vi "MAIN - Car Wash.vi"() -> ()   [LabVIEW 2015, in "Car Wash.lvlib"]
uses:
  Car Wash.lvlib
  Components/State Declaration.ctl
  Components/System Trigger.ctl
  Components/System Trigger Element.ctl
  <vilib>/Utility/error.llb/DialogTypeEnum.ctl
  Components/AMC/Read Termination Message.vi
  Components/AMC/Update Message Routing Info.vi
  Components/AMC/Create Multiple Messages.vi
  Components/AMC/Create Single Message.vi
  Components/TypeDef - SHIFTER.ctl
  Components/AMC/Globals.vi
  Components/AMC/Send Message.vi
  Components/Dependencies.llb/TLB`_Dependencies.lvlib
  Components/AMC/AMC.lvlib
panel:
  out "Status":string
  in  "Start Wash":bool
  in  "Reset Car":bool
  out "Wash Progress":i32(slide) scale=0.0..6.0
  in  "Giant Blowdryers":bool
  in  "Rinse":bool
  in  "Wax":bool
  in  "Roller Brushes":bool
  in  "Soap":bool
  in  "Pre-Soak":bool
  out "error out":errorcluster
  # "Car Wash"
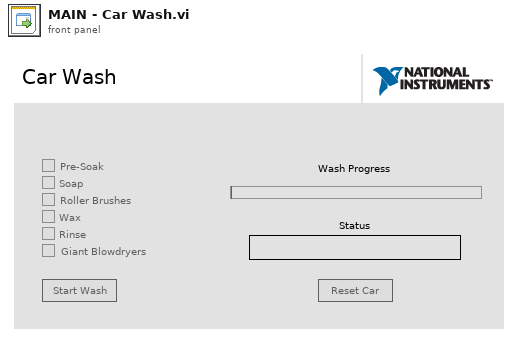
[diagram p1: front panel]
types:
  T1 = typedef "Car Wash.lvlib/System Trigger.ctl" = enum16{"<None>", "Cache User Parameters", "Close Application", "Start Wash", "Reset Car"}
  T2 = typedef "Car Wash.lvlib/State Declaration.ctl" = enum16{"<Startup>", "Idle", "Washing", "<Shutdown>"}
  T3 = enum16{"Clear SR", "Set Display", "Set Shifter", "Initialize Events", "Init Q"}
  T4 = typedef "Car Wash.lvlib/TypeDef - SHIFTER.ctl" = cluster{"State":T2, "User Data":cluster{"Active Item Tag":string, "Pre-Soak":bool, "Soap":bool, "Roller Brushes":bool, "Wax":bool, "Rinse":bool, "Giant Blowdryers":bool}, "Display Data":cluster{"Active Item Tag":string, "Wash Progress":i32, "Status":string}, "User Parameter Controls":refnum<vi>[], "Framework Data":cluster{"Exit Event":T5, "Terminate Error":errorcluster}, "Private Data":cluster{"Active Item Tag":string, "Step Booleans Array":bool[], "Step Names Array":string[], "Wash Done?":bool, "Step Duration":i32}}
  T5 = typedef "Car Wash.lvlib/TLB`_Dependencies.lvlib/Exit Event Ref.ctl" = refnum<user-event>
  T6 = typedef "Car Wash.lvlib/System Trigger Element.ctl" = cluster{"System Triggers":T1, "Trigger Data":variant}
  T7 = typedef "Car Wash.lvlib/AMC.lvlib/Message Queue.ctl" = refnum<queue>
  T8 = enum8{"Enabled", "Disabled", "Disabled and Grayed Out"}
  T9 = typedef "DialogTypeEnum.ctl" = enum16{"no dialog", "OK message", "continue or stop message", "auto error handling dialog", "OK message + warnings", "continue/stop + warnings"}
  T10 = enum32{"Invalid", "Standard", "Closed", "Hidden", "Minimized", "Maximized"}
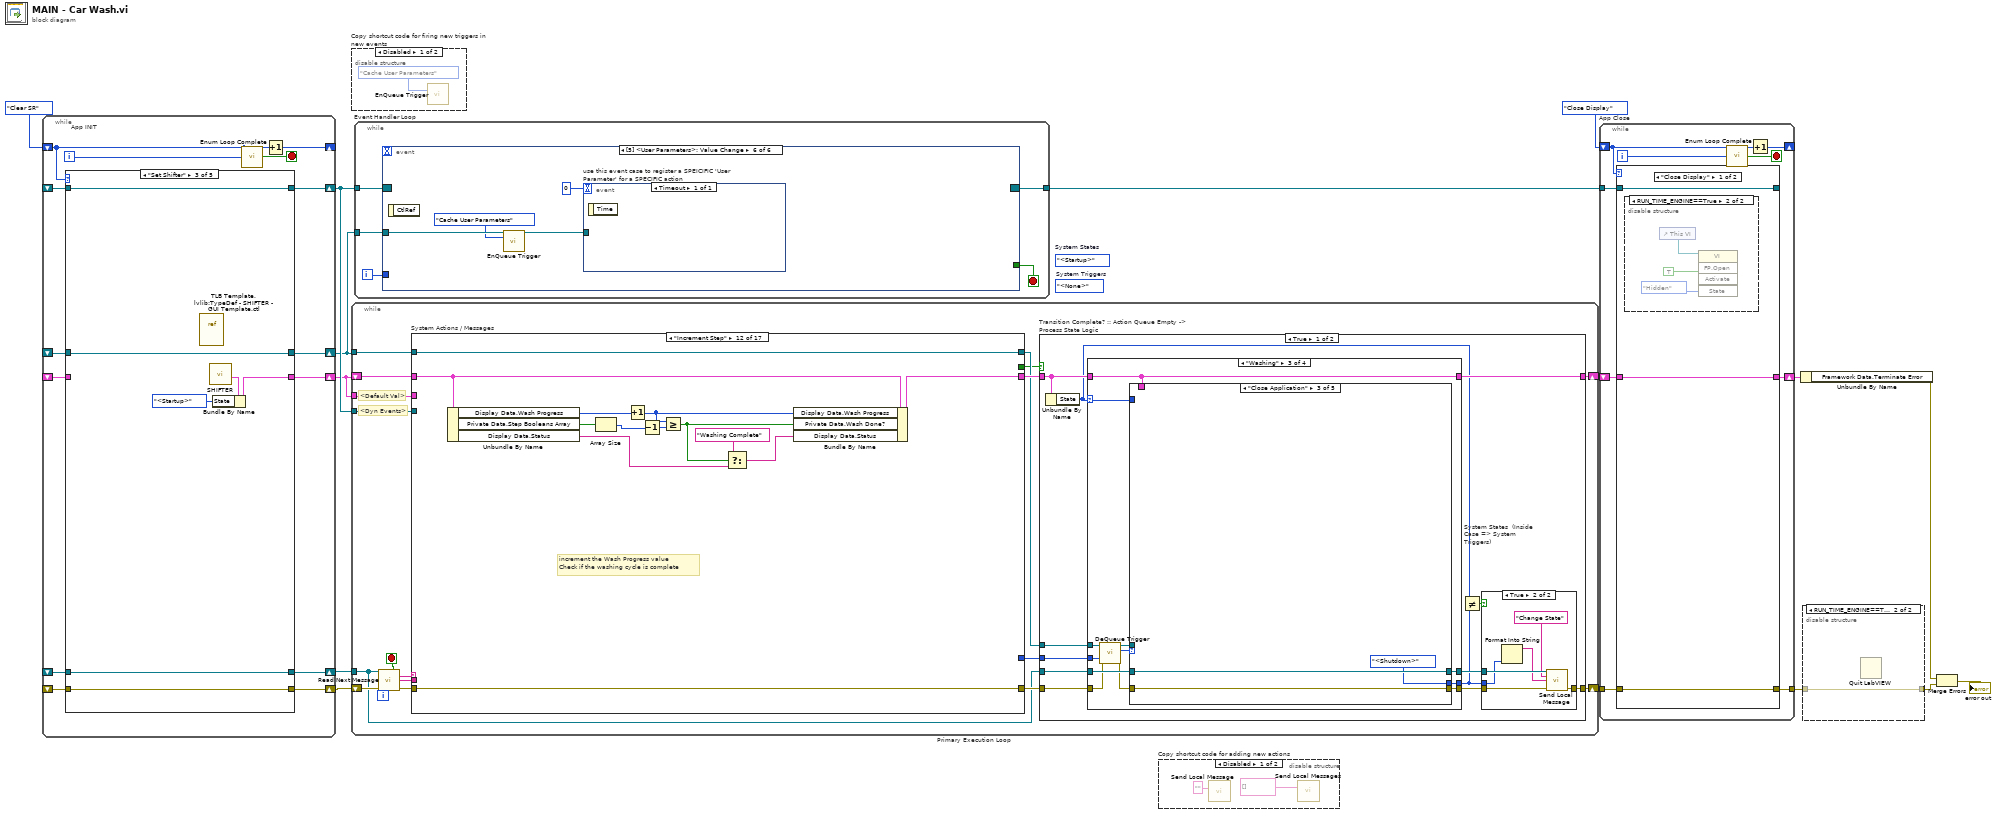
[diagram p0: block diagram]
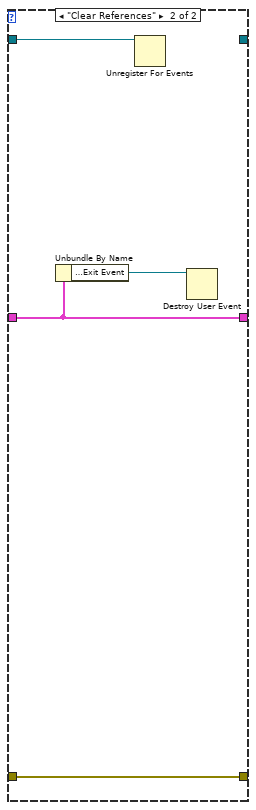
[diagram p6: hidden frame]
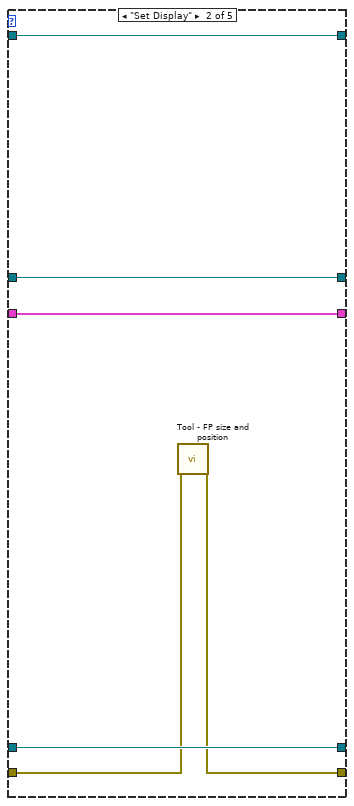
[diagram p8: hidden frame]
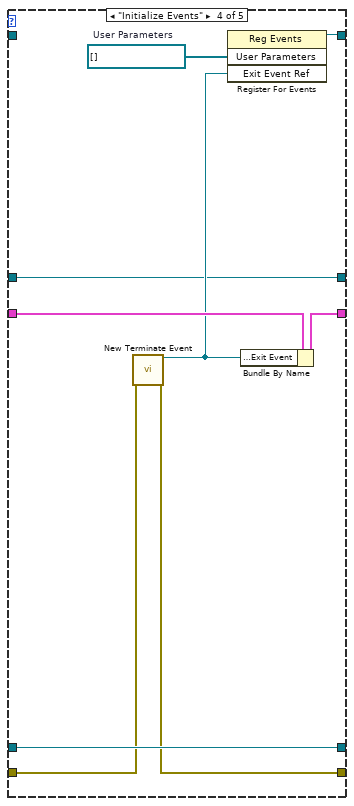
[diagram p9: hidden frame]
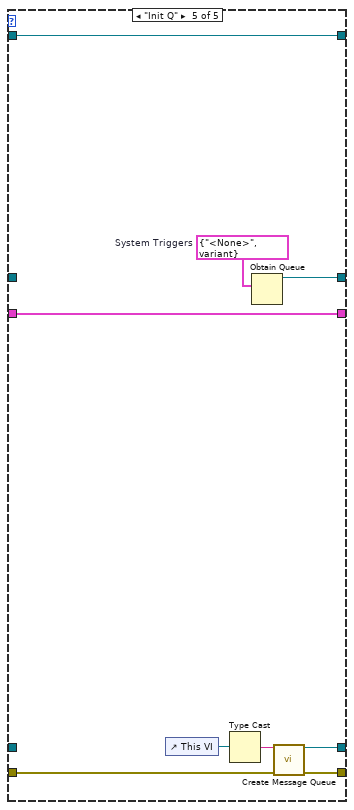
[diagram p10: hidden frame]
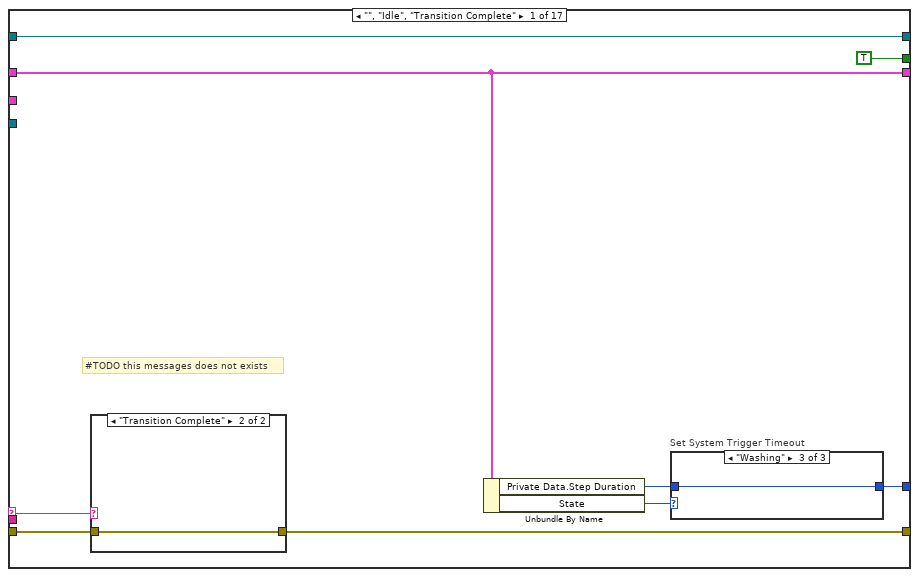
[diagram p11: hidden frame]
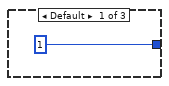
[diagram p13: hidden frame]
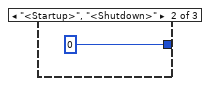
[diagram p14: hidden frame]
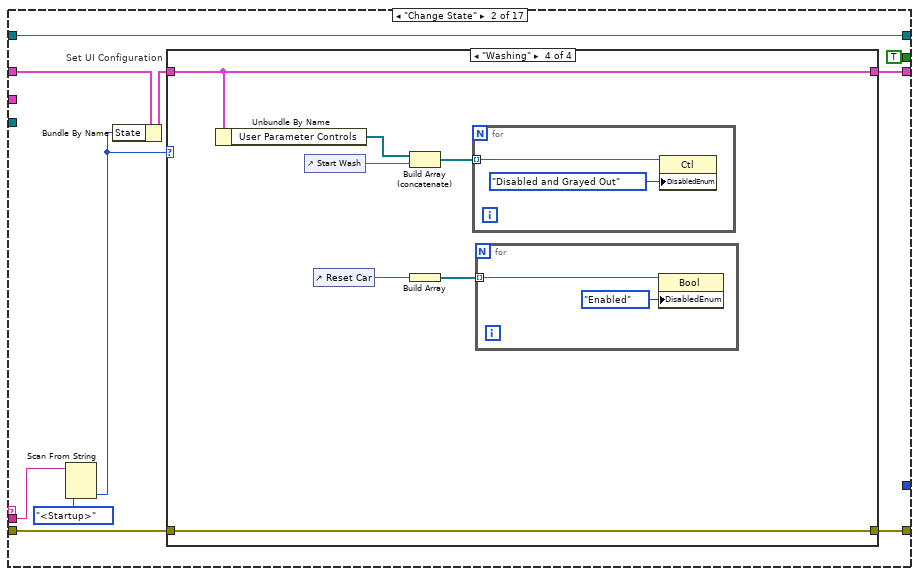
[diagram p15: hidden frame]
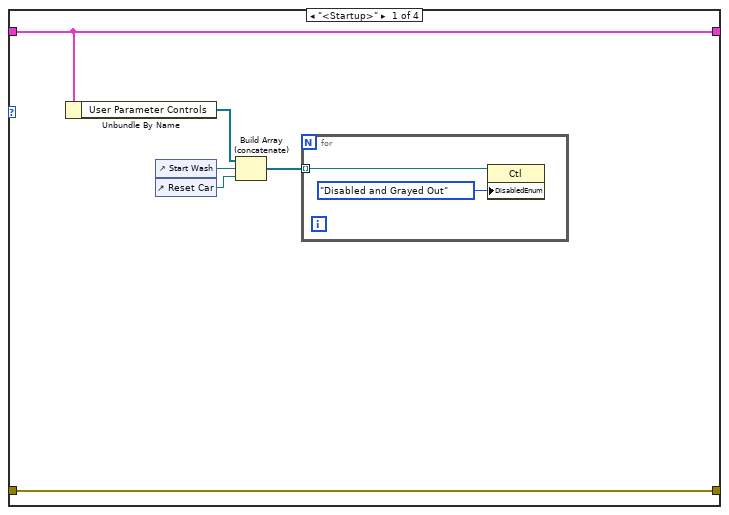
[diagram p16: hidden frame]
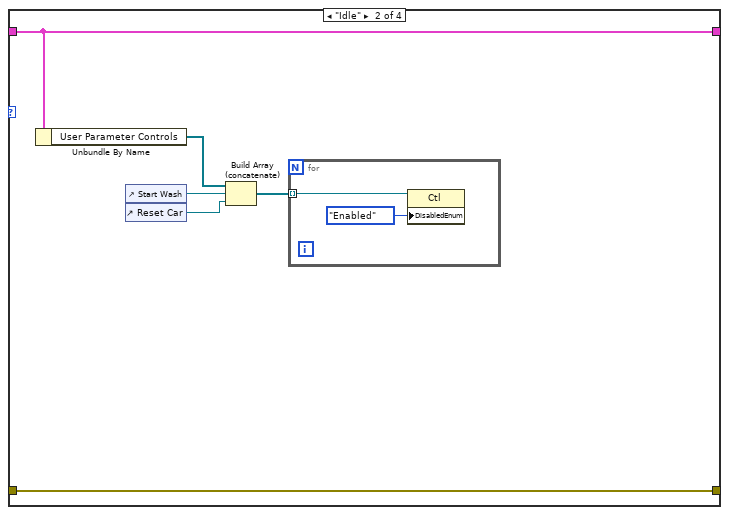
[diagram p17: hidden frame]
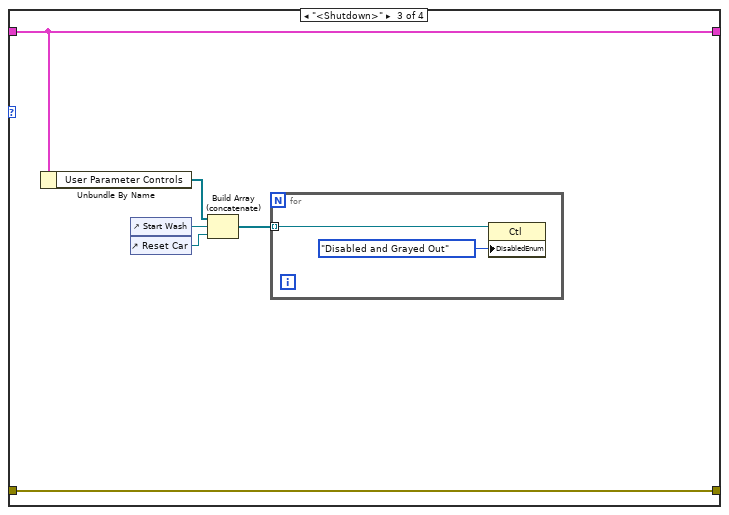
[diagram p18: hidden frame]
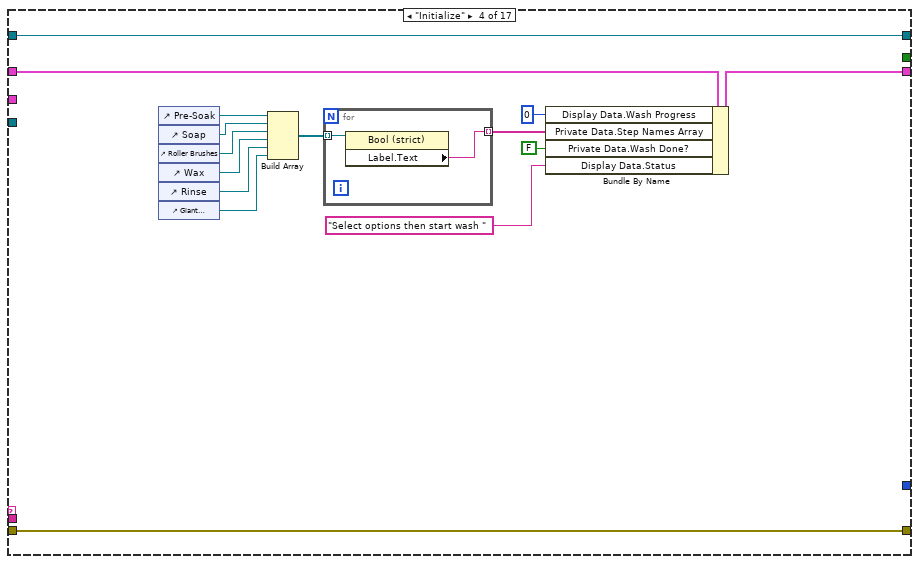
[diagram p20: hidden frame]
diagram:
  (unwired) System_Trigger."<None>"  # System Triggers
  (unwired) State_Declaration."<Startup>"  # System States
  n1 = while "App INIT" {
    shift-right: [w23] -> _
    shift-left: T3."Clear SR" -> [w18]
    shift-right: [w29] -> w9
    shift-left: _ -> [w22]
    shift-right: [w26] -> w8
    shift-left: _ -> [w21]
    shift-right: [w28] -> w11
    shift-left: _ -> [w20]
    shift-right: [w27] -> w1
    shift-left: _ -> [w19]
    shift-right: [w17] -> w2
    shift-left: _ -> [w16]
    i -> [w24]
    stop <- w25 stop-if-true
    n2 = case shown="\"Set Shifter\"" w18 {
      tunnel: [_ w33 w42 w51 w56] -> w29
      tunnel: [_ w31 w41 w44 w55] -> w26
      tunnel: [_ w35 w36 w48 w54] -> w27
      tunnel: [_ w34 w40 w47 w60] -> w28
      tunnel: w22 -> [_ w33 w42 w51 _]
      tunnel: w21 -> [_ w32 w41 w45 w59]
      tunnel: w20 -> [_ w34 w40 _ w60]
      tunnel: w19 -> [_ w35 _ w49 w54]
      tunnel: [_ w30 w39 w43 w58] -> w17
      tunnel: w16 -> [_ w30 w39 w43 _]
      frame "Clear SR" {
      }
      frame "Set Display" {
        n3 = call "Tool - FP size and position.vi"("error in (no error)"=w32) -> ("error out"=w31:errorcluster)  [unwired: 7 in, 11 out]
      }
      frame "Set Shifter" {
        n4 = vi-ref "TLB Template.lvlib:TypeDef - SHIFTER - GUI Template.ctl"() -> ()  [unwired: 1 out]
        n5 = call "SHIFTER.vi"() -> ("SHIFTER DATA"=w37:T4)  [unwired: 15 in]
        n6 = Bundle By Name(cluster=w37, "State"=State_Declaration."<Startup>") -> (w36:T4)
      }
      frame "Initialize Events" {
        w50 = refnum<vi>[] []  # User Parameters
        n7 = call "New Terminate Event.vi"("error in (no error)"=w45) -> ("Exit Event Ref"=w46:T5, "error out"=w44:errorcluster)  [unwired: 13 in]
        n8 = register-events(w50, w46) -> (reference out=w47:refnum<event-registration>)  [unwired: 2 in, 1 out]
        n9 = Bundle By Name(cluster=w49, "Framework Data.Exit Event"=w46) -> (w48:T4)
      }
      frame "Init Q" {
        w57 = T6 {"System Triggers"=enum."<None>", "Trigger Data"=variant}  # System Triggers
        n10 = control-ref of="This VI"() -> (w53:refnum<vi>)
        n11 = Type Cast(x=w53) -> (*(type *) &x=w52:string)  [unwired: 1 in]
        n12 = Obtain Queue(element data type=w57) -> (queue out=w58:refnum<queue>)  [unwired: 4 in, 2 out]
        n13 = call "Create Message Queue.vi"("message queue name"=w52, "error in"=w59) -> ("message queue out"=w56:T7, "error out"=w55:errorcluster)  [unwired: 12 in]
      }
    }
    n14 = call "Enum Loop Complete.vi"("Current State Enum"=w18, "Itteration"=w24) -> ("Loop Complete?"=w25:bool)  [unwired: 13 out]
    n15 = Increment(x=w18) -> (x+1=w23:T3)
  }
  n16 = disable-structure "Copy shortcut code for firing new triggers in new events" shown="Disabled" {
    frame Disabled {
      n17 = call "EnQueue Trigger.vi"("System Triggers"=System_Trigger."Cache User Parameters") -> ()  [unwired: 13 in, 2 out]
    }
    frame Enabled {
    }
  }
  n18 = while "Primary Execution Loop" {
    shift-right: [w68] -> w15
    shift-left: w8 -> [w75]
    shift-right: [w71] -> w14
    shift-left: w1 -> [w78]
    tunnel: w1 -> [w77]
    tunnel: w9 -> [w66]
    tunnel: w11 -> [w76]
    tunnel: w2 -> [w67]
    stop <- w73 stop-if-true
    # "<Dyn Events>"
    # "<Default Val>"
    n19 = call "Read Next Message.vi"("message queue in"=w66, "error in"=w75) -> ("exit process?"=w73:bool, "message name"=w72:string, "message value"=w63:string, "error out"=w74:errorcluster)  [unwired: 6 in, 4 out]
    n20 = case "System Actions / Messages" shown="\"Increment Step\"" w72 {
      selector: w72 -> [w82 _ _ _ _ _ _ _ _ _ _ _ _ _ _ _ w270]
      tunnel: [w81 w97 w140 w154 w169 w180 w183 w191 w198 w201 w212 w229 w233 w236 w241 w264 w274] -> w69
      tunnel: w74 -> [w80 w96 w140 w154 w169 w180 w183 w191 w198 w201 w212 w229 w233 w236 w242 w263 w275]
      tunnel: w78 -> [w83 w93 w139 w150 w168 w173 w182 w193 w196 w199 w205 w225 w231 w235 w239 w267 w276]
      tunnel: w77 -> [_ _ _ _ _ _ _ _ _ _ _ _ _ _ _ _ _]
      tunnel: [w83 w95 w139 w153 w167 w172 w182 w192 w196 w199 w204 w227 w231 w235 w240 w267 w276] -> w70
      tunnel: [w84 _ _ _ _ _ _ _ _ _ _ _ w230 _ _ _ _] -> w62
      tunnel: w76 -> [_ _ _ _ w166 _ _ _ _ _ _ _ _ _ _ _ _]
      tunnel: [w86 w101 w138 w155 w165 w179 w181 w190 w197 w200 w211 w228 w232 w234 w237 w261 w268] -> w65
      tunnel: w67 -> [w86 w101 w138 w155 w165 w179 w181 w190 w197 w200 w211 w228 w232 w234 w237 w261 w268]
      tunnel: [TRUE TRUE _ _ _ _ _ _ _ _ _ _ _ _ _ _ _] -> w64
      tunnel: w63 -> [_ w100 _ _ _ _ _ _ _ _ _ _ _ _ _ _ _]
      frame "", "Idle", "Transition Complete" {
        # "#TODO this messages does not exists"
        n21 = case shown="\"Transition Complete\"" w82 {
          tunnel: [w88 w89] -> w81
          tunnel: w80 -> [w88 w89]
          frame Default {
          }
          frame "Transition Complete" {
          }
        }
        n22 = Unbundle By Name(w83) -> ("Private Data.Step Duration"=w79:i32, "State"=w85:T2)
        n23 = case "Set System Trigger Timeout" shown="\"Washing\"" w85 {
          tunnel: [1 0 w92] -> w84
          tunnel: w79 -> [_ _ w92]
          frame Default {
          }
          frame "<Startup>", "<Shutdown>" {
          }
          frame "Washing" {
          }
        }
      }
      frame "Change State" {
        n24 = Scan From String(input string=w100, default 1=State_Declaration."<Startup>" ("State")) -> (output 1=w98:T2)  [unwired: 3 in, 3 out]
        n25 = Bundle By Name(cluster=w93, "State"=w98) -> (w94:T4)
        n26 = case "Set UI Configuration" shown="\"Washing\"" w98 {
          tunnel: [w108 w116 w124 w133] -> w97
          tunnel: w96 -> [w108 w116 w124 w133]
          tunnel: [w104 w112 w120 w128] -> w95
          tunnel: w94 -> [w104 w112 w120 w128]
          frame "<Startup>" {
            n27 = Unbundle By Name(w104) -> ("User Parameter Controls"=w103:refnum<vi>[])
            n28 = control-ref of="Start Wash"() -> (w107:refnum<vi>)
            n29 = control-ref of="Reset Car"() -> (w105:refnum<vi>)
            n30 = Build Array (concatenate)(w103, w107, w105) -> (w106:refnum<vi>[])
            n31 = for {
              tunnel: w106 -> [w110] mode=indexing
              n32 = property class="Ctl"(reference=w110, "DisabledEnum"=T8."Disabled and Grayed Out" ("Disabled")) -> ()  [unwired: 1 in, 2 out]
            }
          }
          frame "Idle" {
            n33 = Unbundle By Name(w112) -> ("User Parameter Controls"=w111:refnum<vi>[])
            n34 = control-ref of="Start Wash"() -> (w114:refnum<vi>)
            n35 = control-ref of="Reset Car"() -> (w113:refnum<vi>)
            n36 = Build Array (concatenate)(w111, w114, w113) -> (w115:refnum<vi>[])
            n37 = for {
              tunnel: w115 -> [w118] mode=indexing
              n38 = property class="Ctl"(reference=w118, "DisabledEnum"=T8."Enabled" ("Disabled")) -> ()  [unwired: 1 in, 2 out]
            }
          }
          frame "<Shutdown>" {
            n39 = Unbundle By Name(w120) -> ("User Parameter Controls"=w119:refnum<vi>[])
            n40 = control-ref of="Start Wash"() -> (w122:refnum<vi>)
            n41 = control-ref of="Reset Car"() -> (w121:refnum<vi>)
            n42 = Build Array (concatenate)(w119, w122, w121) -> (w123:refnum<vi>[])
            n43 = for {
              tunnel: w123 -> [w126] mode=indexing
              n44 = property class="Ctl"(reference=w126, "DisabledEnum"=T8."Disabled and Grayed Out" ("Disabled")) -> ()  [unwired: 1 in, 2 out]
            }
          }
          frame "Washing" {
            n45 = Unbundle By Name(w128) -> ("User Parameter Controls"=w127:refnum<vi>[])
            n46 = control-ref of="Start Wash"() -> (w131:refnum<vi>)
            n47 = control-ref of="Reset Car"() -> (w129:refnum<vi>)
            n48 = Build Array (concatenate)(w127, w131) -> (w132:refnum<vi>[])
            n49 = Build Array(w129) -> (w130:refnum<vi>[])
            n50 = for {
              tunnel: w132 -> [w137] mode=indexing
              n51 = property class="Ctl"(reference=w137, "DisabledEnum"=T8."Disabled and Grayed Out" ("Disabled")) -> ()  [unwired: 1 in, 2 out]
            }
            n52 = for {
              tunnel: w130 -> [w135] mode=indexing
              n53 = property class="Bool"(reference=w135, "DisabledEnum"=T8."Enabled" ("Disabled")) -> ()  [unwired: 1 in, 2 out]
            }
          }
        }
      }
      frame "/*********Initialize********/" {
      }
      frame "Initialize" {
        n54 = control-ref of="Pre-Soak"() -> (w147:refnum<vi>)
        n55 = control-ref of="Soap"() -> (w146:refnum<vi>)
        n56 = control-ref of="Roller Brushes"() -> (w145:refnum<vi>)
        n57 = control-ref of="Wax"() -> (w144:refnum<vi>)
        n58 = control-ref of="Rinse"() -> (w143:refnum<vi>)
        n59 = control-ref of="Giant Blowdryers"() -> (w142:refnum<vi>)
        n60 = Build Array(w147, w146, w145, w144, w143, w142) -> (w148:refnum<vi>[])
        n61 = for {
          tunnel: w148 -> [w156] mode=indexing
          tunnel: [w157] -> w149 mode=indexing
          n62 = property class="Bool (strict)"(reference=w156) -> ("Label.Text"=w157:string)  [unwired: 1 in, 2 out]
        }
        n63 = Bundle By Name(cluster=w150, "Display Data.Wash Progress"=0, "Private Data.Step Names Array"=w149, "Private Data.Wash Done?"=FALSE, "Display Data.Status"="Select options then start wash " ("Status")) -> (w153:T4)
      }
      frame "Register User Parameters" {
        n64 = control-ref of="Giant Blowdryers"() -> (w164:refnum<vi>)
        n65 = control-ref of="Rinse"() -> (w159:refnum<vi>)
        n66 = control-ref of="Wax"() -> (w160:refnum<vi>)
        n67 = control-ref of="Roller Brushes"() -> (w161:refnum<vi>)
        n68 = control-ref of="Soap"() -> (w162:refnum<vi>)
        n69 = control-ref of="Pre-Soak"() -> (w163:refnum<vi>)
        n70 = Build Array(w164, w159, w160, w161, w162, w163) -> (w158:refnum<vi>[])
        n71 = register-events(reference=w166, w158) -> ()  [unwired: 2 in, 2 out]
        n72 = Bundle By Name(cluster=w168, "User Parameter Controls"=w158) -> (w167:T4)
      }
      frame "Create Steps Array" {
        # "This action pushes the current value of the wash options to the Step Booleans Array"
        n73 = Unbundle By Name(w173) -> ("User Data.Pre-Soak"=w170:bool, "User Data.Soap"=w178:bool, "User Data.Roller Brushes"=w177:bool, "User Data.Wax"=w176:bool, "User Data.Rinse"=w175:bool, "User Data.Giant Blowdryers"=w174:bool)
        n74 = Build Array(w170, w178, w177, w176, w175, w174) -> (w171:bool[])
        n75 = Bundle By Name(cluster=w173, "Private Data.Step Booleans Array"=w171) -> (w172:T4)
      }
      frame "/*********Display Updates********/" {
      }
      frame "Cache User Parameters" {
        # "This Action reads the control values and places the data into the Mother Cluster"
        n76 = Bundle By Name(cluster=w193, "User Data.Pre-Soak"="Pre-Soak", "User Data.Soap"="Soap", "User Data.Roller Brushes"="Roller Brushes", "User Data.Wax"="Wax", "User Data.Rinse"="Rinse", "User Data.Giant Blowdryers"="Giant Blowdryers") -> (w192:T4)
      }
      frame "Update Display" {
        n77 = Unbundle By Name(w196) -> ("Display Data.Wash Progress"=→"Wash Progress":i32, "Display Data.Status"=→"Status":string)
      }
      frame "/*********Primary Execution********/" {
      }
      frame "Evaluate Step" {
        n78 = Unbundle By Name(w205) -> ("Display Data.Wash Progress"=w208:i32, "Private Data.Step Booleans Array"=w210:bool[], "Private Data.Step Names Array"=w209:string[])
        n79 = Index Array(array=w209, index=w208) -> (element=w207:string)
        n80 = Index Array(array=w210, index=w208) -> (element=w206:bool)
        n81 = case shown="False" w206 {
          tunnel: w207 -> [_ w216]
          tunnel: ["" ("String") w216] -> w203
          tunnel: [0 ("Private Data.Step Duration") 1000 ("Private Data.Step Duration")] -> w202
          frame False {
            # "Do nothing\ndo not execute the wash option\ndo not update the status"
          }
          frame True {
          }
        }
        n82 = Bundle By Name(cluster=w205, "Private Data.Step Duration"=w202, "Display Data.Status"=w203) -> (w204:T4)
      }
      frame "Increment Step" {
        # "increment the Wash Progress value\nCheck if the washing cycle is complete"
        n83 = Unbundle By Name(w225) -> ("Display Data.Wash Progress"=w223:i32, "Private Data.Step Booleans Array"=w224:bool[], "Display Data.Status"=w217:string)
        n84 = Array Size(array=w224) -> (size(s)=w226:i32)
        n85 = Increment(x=w223) -> (x+1=w222:i32)
        n86 = Decrement(x=w226) -> (x-1=w221:i32)
        n87 = Greater Or Equal?(x=w222, y=w221) -> (x >= y?=w219:bool)
        n88 = Select(t="Washing Complete", s=w219, f=w217) -> (s? t:f=w218:string)
        n89 = Bundle By Name(cluster=w225, "Display Data.Wash Progress"=w222, "Private Data.Wash Done?"=w219, "Display Data.Status"=w218) -> (w227:T4)
      }
      frame "Set Step Duration" {
        # "This action needs to be called last so that\nthe timeout is triggered. A timeout is triggered\nafter x ms without a system trigger."
        n90 = Unbundle By Name(w231) -> ("Private Data.Step Duration"=w230:i32)
      }
      frame "/*********Shutdown********/" {
      }
      frame "Error" {
        n91 = Unbundle By Name(w239) -> ("State"=w238:T2)
        n92 = case shown="Default" w238 {
          tunnel: w242 -> [w250]
          tunnel: [w249] -> w241
          tunnel: w239 -> [w246]
          tunnel: [w245] -> w240
          tunnel: w237 -> [w243]
          frame Default {
            n93 = call <vilib>:"General Error Handler CORE.vi"("type of dialog (OK msg:1)"=DialogTypeEnum."auto error handling dialog", "error in (no error)"=w250) -> ("stop event propagated"=w248:bool, "error out"=w244:errorcluster)  [unwired: 12 out]
            n94 = case "User Chose to Stop and Not Continue\nFALSE = Continue: CLEAR ERRORS" shown="False" w248 {
              tunnel: [w251 w256] -> w249
              tunnel: w244 -> [w252 w258]
              tunnel: w246 -> [w253 w260]
              tunnel: [w253 w259] -> w245
              tunnel: w243 -> [_ w257]
              frame False {
                n95 = call <vilib>:"Clear Errors.vi"("error in (no error)"=w252) -> ("error out"=w251:errorcluster)  [unwired: 1 in, 5 out]
              }
              frame True {
                n96 = call <vilib>:"Clear Errors.vi"("error in (no error)"=w258) -> ("error out"=w255:errorcluster)  [unwired: 1 in, 5 out]
                n97 = Bundle By Name(cluster=w260, "Framework Data.Terminate Error"=w258) -> (w259:T4)
                n98 = call "EnQueue Trigger.vi"("Queue in"=w257, "System Triggers"=System_Trigger."Close Application", "error in (no error)"=w255) -> ("error out"=w256:errorcluster)  [unwired: 11 in, 1 out]
              }
            }
          }
        }
      }
      frame "Exit" {
        w262 = refnum<class> refnum  # event data
        # "Don't wire 'Error In'\nMust Execute Regardless"
        n99 = Unbundle By Name(w267) -> ("Framework Data.Exit Event"=w266:T5)  [unwired: 1 out]
        n100 = Generate User Event(user event=w266, event data cluster=w262) -> (error out=w265:errorcluster)  [unwired: 2 in, 1 out]
        n101 = Merge Errors(w265, w263) -> (w264:errorcluster)
      }
      frame Default {
        w272 = 1 items=["No error", "Argument error", "Memory is full", "Out of zone", "End of file", "File already open", "Generic file I/O error", "File not found", "File permission error", "Disk is full", "Duplicate path", "Too many files open", "System feature not enabled", "Resource file not found", "Cannot add resource", "Resource not found", "Image not found", "Image memory error", "Pen does not exist", "Config type invalid", "Config token not found", "Config parse error", "Config memory error", "Bad external code format", "Bad external code offset", "External code not present", "Null window", "Destroy window error", "Null menu", "Print aborted", "Bad print record", "Print driver error", "Windows error during printing", "Memory error during printing", "Print dialog error", "Generic print error", "Invalid device refnum", "Device not found", "Device parameter error", "Device unit error", "Cannot open device", "Device call aborted", "Generic error", "Cancelled by user", "Object ID too low", "Object ID too high", "Object not in heap", "Unknown heap", "Unknown object (invalid DefProc)", "Unknown object (DefProc not in table)", "Message out of range", "Invalid (null) method", "Unknown message", "Manager call not supported", "Bad address", "Network operation in progress", "Network operation timed out", "Connection is busy", "Network attribute not supported", "Network error", "Address in use", "System out of memory", "Connection aborted", "Connection refused", "Not connected", "Already connected", "Connection closed", "Initialization error (interapplication manager)", "Bad occurrence", "Wait on unbound occurrence handler", "Occurrence queue overflow", "Datalog type conflict", "Unused", "Unrecognized type (interapplication manager)", "Memory corrupt", "Failed to make temporary DLL", "Old CIN version", "Drag socket not found", "Failed to load drop-object", "Failed to register OLE object", "Failed to release OLE object", "Format specifier type mismatch", "Unknown format specifier", "Too few format specifiers", "Too many format specifiers", "Scan failed", "Newer CIN version", "Error converting to variant", "Runtime menu error", "Password tampered", "Variant attribute not found", "Incompatible variant data type", "Event data is not available", "Event Store is not present", "Occurrence is not found", "Event Queue is not created", "Event info is not available", "Refnum passed is NULL", "Error retrieving Class GUID", "Error retrieving CoClass GUID", "Error retrieving TypeLib GUID.", "Bad built application magic bytes.", "Specific driver is different from the specific driver associated with the Logical Name.", "There is no session opened to the class driver.", "Max Error", "MAX - Error with config objects", "MAX - Error loading configuration", "MAX - Group not supported"]
        w273 = TRUE  # status
        n102 = Format Into String(format string="DEVELOPER ERROR:\nImproper Action Requested\n================\nAction {%s} does not exist within this architecture\n\nCheck for spelling and case errors" ("source"), w270) -> (resulting string=w271:string)  [unwired: 2 in, 1 out]
        n103 = Bundle By Name(cluster=w275, "status"=w273, "code"=w272, "source"=w271) -> (w274:errorcluster)
      }
    }
    n104 = case "Transition Complete? :: Action Queue Empty -> Process State Logic" shown="True" w64 {
      tunnel: [w288 w410] -> w71
      tunnel: w70 -> [w278 w410]
      tunnel: w69 -> [w287 w409]
      tunnel: w66 -> [w286 _]
      tunnel: [w282 w409] -> w68
      tunnel: w65 -> [w285 _]
      tunnel: w62 -> [w279 _]
      frame True {
        n105 = Unbundle By Name(w278) -> ("State"=w277:T2)
        n106 = case "System States  (Inside Case => System Triggers)" shown="\"Washing\"" w277 {
          selector: w277 -> [_ w317 w357 _]
          tunnel: [w304 w323 w352 w400] -> w288
          tunnel: w278 -> [w304 w323 w352 w400]
          tunnel: w287 -> [w298 w315 w355 w394]
          tunnel: w286 -> [w296 w319 w359 w392]
          tunnel: [w303 w322 w362 w399] -> w283
          tunnel: w285 -> [w306 w324 w363 w402]
          tunnel: [w302 w321 w361 w398] -> w284
          tunnel: [w301 w320 w360 w397] -> w281
          tunnel: w279 -> [w300 w313 w353 w396]
          frame "<Startup>" {
            n107 = call "DeQueue Trigger.vi"("Queue in"=w306, "Timeout (0)"=w300, "error in (no error)"=w298) -> ("Queue out"=w299:refnum<queue>, "System Triggers"=w305:T1, "error out"=w297:errorcluster)  [unwired: 9 in, 1 out]
            n108 = case shown="\"<None>\", Default" w305 {
              tunnel: w304 -> [_]
              tunnel: [w310] -> w303
              tunnel: w297 -> [w311]
              tunnel: w296 -> [w309]
              tunnel: [w308] -> w302
              tunnel: [State_Declaration."Idle" ("State")] -> w301
              tunnel: w299 -> [_]
              frame "<None>", Default {
                w307 = string[] ["Initialize", "Cache User Parameters", "Register User Parameters", "Update Display"]  # Initial Elements
                n109 = call "Send Local Messages.vi"("message queue in"=w309, "message names"=w307, "error in"=w311) -> ("message queue out"=w308:T7, "error out"=w310:errorcluster)  [unwired: 10 in, 1 out]
              }
            }
          }
          frame "Idle" {
            n110 = call "DeQueue Trigger.vi"("Queue in"=w324, "Timeout (0)"=w313, "error in (no error)"=w315) -> ("Queue out"=w318:refnum<queue>, "System Triggers"=w316:T1, "error out"=w314:errorcluster)  [unwired: 9 in, 1 out]
            n111 = case shown="\"Start Wash\"" w316 {
              tunnel: w323 -> [_ _ _ _ _ _]
              tunnel: [w325 w329 w333 w338 w340 w346] -> w322
              tunnel: w314 -> [w325 w329 w336 w338 w343 w349]
              tunnel: w319 -> [w326 w330 w335 w339 w341 w347]
              tunnel: [w326 w330 w334 w339 w342 w348] -> w321
              tunnel: [State_Declaration."Idle" ("State") State_Declaration."<Shutdown>" ("State") w331 State_Declaration."Idle" ("State") State_Declaration."Washing" ("State") State_Declaration."Idle" ("State")] -> w320
              tunnel: w318 -> [_ _ _ _ _ _]
              tunnel: w317 -> [_ _ w331 _ _ _]
              frame "<None>" {
              }
              frame "Close Application" {
              }
              frame "Cache User Parameters" {
                n112 = call "Send Local Message.vi"("message queue in"=w335, "message name"="Cache User Parameters" ("Message Name"), "error in"=w336) -> ("message queue out"=w334:T7, "error out"=w333:errorcluster)  [unwired: 10 in, 1 out]
              }
              frame Default {
              }
              frame "Start Wash" {
                # "next state to go to"
                # "Actions to perform"
                n113 = call "Send Local Messages.vi"("message queue in"=w341, "message names"=string[] ["Initialize", "Update Display", "Create Steps Array"], "error in"=w343) -> ("message queue out"=w342:T7, "error out"=w340:errorcluster)  [unwired: 10 in, 1 out]
              }
              frame "Reset Car" {
                # "Next State"
                # "Actions to perform"
                n114 = call "Send Local Messages.vi"("message queue in"=w347, "message names"=string[] ["Initialize", "Update Display"], "error in"=w349) -> ("message queue out"=w348:T7, "error out"=w346:errorcluster)  [unwired: 10 in, 1 out]
              }
            }
          }
          frame "Washing" {
            n115 = call "DeQueue Trigger.vi"("Queue in"=w363, "Timeout (0)"=w353, "error in (no error)"=w355) -> ("Queue out"=w358:refnum<queue>, "System Triggers"=w356:T1, "error out"=w354:errorcluster)  [unwired: 9 in, 1 out]
            n116 = case shown="\"Close Application\"" w356 {
              tunnel: w352 -> [w369 _ _ _ _]
              tunnel: [w372 w378 w381 w385 w390] -> w362
              tunnel: w354 -> [w373 w379 w381 w388 w390]
              tunnel: w359 -> [w371 w377 w382 w387 w391]
              tunnel: [w370 w376 w382 w386 w391] -> w361
              tunnel: [w366 State_Declaration."Idle" ("State") State_Declaration."<Shutdown>" ("State") w383 State_Declaration."Washing" ("State")] -> w360
              tunnel: w358 -> [_ _ _ _ _]
              tunnel: w357 -> [_ _ _ w383 _]
              frame "<None>" {
                # "Conditional next state"
                # "action list"
                n117 = Unbundle By Name(w369) -> ("Private Data.Wash Done?"=w365:bool)
                n118 = call "Send Local Messages.vi"("message queue in"=w371, "message names"=string[] ["Evaluate Step", "Increment Step", "Update Display"], "error in"=w373) -> ("message queue out"=w370:T7, "error out"=w372:errorcluster)  [unwired: 10 in, 1 out]
                n119 = Select(t=State_Declaration."Idle" ("State"), s=w365, f=State_Declaration."Washing" ("State")) -> (s? t:f=w366:T2)
              }
              frame "Reset Car" {
                n120 = call "Send Local Messages.vi"("message queue in"=w377, "message names"=string[] ["Initialize", "Update Display"], "error in"=w379) -> ("message queue out"=w376:T7, "error out"=w378:errorcluster)  [unwired: 10 in, 1 out]
              }
              frame "Close Application" {
              }
              frame "Cache User Parameters" {
                n121 = call "Send Local Message.vi"("message queue in"=w387, "message name"="Cache User Parameters" ("Message Name"), "error in"=w388) -> ("message queue out"=w386:T7, "error out"=w385:errorcluster)  [unwired: 10 in, 1 out]
              }
              frame Default {
              }
            }
          }
          frame "<Shutdown>" {
            n122 = call "DeQueue Trigger.vi"("Queue in"=w402, "Timeout (0)"=w396, "error in (no error)"=w394) -> ("Queue out"=w395:refnum<queue>, "System Triggers"=w401:T1, "error out"=w393:errorcluster)  [unwired: 9 in, 1 out]
            n123 = case shown="\"<None>\", Default" w401 {
              tunnel: w400 -> [_]
              tunnel: [w403] -> w399
              tunnel: w393 -> [w405]
              tunnel: w392 -> [w406]
              tunnel: [w404] -> w398
              tunnel: [State_Declaration."<Shutdown>" ("State")] -> w397
              tunnel: w395 -> [_]
              frame "<None>", Default {
                n124 = call "Send Local Messages.vi"("message queue in"=w406, "message names"=string[] ["Exit"], "error in"=w405) -> ("message queue out"=w404:T7, "error out"=w403:errorcluster)  [unwired: 10 in, 1 out]
              }
            }
          }
        }
        n125 = Not Equal?(x=w277, y=w281) -> (x != y?=w280:bool)
        n126 = case shown="True" w280 {
          tunnel: w284 -> [_ w295]
          tunnel: w283 -> [w289 w294]
          tunnel: [w289 w293] -> w282
          tunnel: w281 -> [_ w291]
          frame False {
          }
          frame True {
            n127 = Format Into String(w291) -> (resulting string=w290:string)  [unwired: 3 in, 1 out]
            n128 = call "Send Local Message.vi"("message queue in"=w295, "message name"="Change State" ("Message Name"), "message value"=w290, "error in"=w294) -> ("error out"=w293:errorcluster)  [unwired: 9 in, 2 out]
          }
        }
      }
      frame False {
      }
    }
  }
  n129 = while "Event Handler Loop" {
    tunnel: w11 -> [w414]
    tunnel: [w413] -> w13
    tunnel: w2 -> [w411]
    i -> [w412]
    stop <- w415 stop-if-true
    n130 = event shown="[5] <User Parameters>: Value Change" {
      selector: w414 -> [_ _ _ _ _ _]
      dyn-events: [_ _ _ _ _ _] -> w413
      timeout: _ -> [_ _ _ _ _ _]
      tunnel: [_ _ _ _ TRUE ("NewVal") _] -> w415
      tunnel: w412 -> [_ _ _ _ _ _]
      tunnel: w411 -> [w417 w420 w422 _ w433 w437]
      event Panel Close? {
        w418 = TRUE  # Discard?
        n131 = event-data() -> ()  [unwired: 2 out]
        n132 = call "EnQueue Trigger.vi"("Queue in"=w417, "System Triggers"=System_Trigger."Close Application") -> ()  [unwired: 12 in, 2 out]
        n133 = event-data("Discard?"=w418) -> ()  [unwired: 1 in, 1 out]
      }
      event "Start Wash": Value Change {
        n134 = event-data() -> ()  [unwired: 4 out]
        n135 = call "EnQueue Trigger.vi"("Queue in"=w420, "System Triggers"=System_Trigger."Start Wash") -> ()  [unwired: 12 in, 2 out]
      }
      event "Reset Car": Value Change {
        n136 = event-data() -> ()  [unwired: 4 out]
        n137 = call "EnQueue Trigger.vi"("Queue in"=w422, "System Triggers"=System_Trigger."Reset Car") -> ()  [unwired: 12 in, 2 out]
      }
      event Mouse Down {
        n138 = event-data() -> ("Button"=w427:u16, "Mods"=w428:cluster{"Double Click":bool, "Menu Key":bool})  [unwired: 1 out]
        n139 = Unbundle By Name(w428) -> ("Double Click"=w424:bool)
        n140 = Equal?(x=u16 2, y=w427) -> (x = y?=w425:bool)
        n141 = And(x=w425, y=w424) -> (x .and. y?=w423:bool)
        n142 = case "Toggle Menu Visibility :: double RIGHT click on logo" shown="True" w423 {
          frame False {
          }
          frame True {
            n143 = property class="VI"() -> (reference out=w431:refnum<vi>, "TB.Visible"=w429:bool)  [unwired: 2 in, 1 out]
            n144 = Not(x=w429) -> (.not. x?=w430:bool)
            n145 = property class="VI"(reference=w431, "TB.Visible"=w430) -> ()  [unwired: 1 in, 2 out]
          }
        }
      }
      event User Event {
        n146 = event-data() -> ()  [unwired: 2 out]
        n147 = call "EnQueue Trigger.vi"("Queue in"=w433, "System Triggers"=System_Trigger."Close Application") -> ()  [unwired: 12 in, 2 out]
      }
      event Value Change {
        n148 = event-data() -> ()  [unwired: 2 out]
        n149 = call "EnQueue Trigger.vi"("Queue in"=w437, "System Triggers"=System_Trigger."Cache User Parameters") -> ("Queue out"=w436:refnum<queue>)  [unwired: 12 in, 1 out]
        n150 = event "use this event case to register a SPEICIFIC 'User Parameter' for a SPECIFIC action" shown="[0] Timeout" {
          selector: _ -> [_]
          dyn-events: _ -> [_]
          timeout: 0 -> [_]
          tunnel: w436 -> [_]
          event Timeout {
            n151 = event-data() -> ()  [unwired: 1 in, 1 out]
          }
        }
      }
    }
  }
  n152 = disable-structure "Copy shortcut code for adding new actions" shown="Disabled" {
    frame Disabled {
      n153 = call "Send Local Message.vi"("message name"="") -> ()  [unwired: 12 in, 3 out]
      n154 = call "Send Local Messages.vi"("message names"=string[] []) -> ()  [unwired: 12 in, 3 out]
    }
    frame Enabled {
    }
  }
  n155 = while "App Close" {
    shift-right: [w447] -> _
    shift-left: enum16{"Close Display", "Clear References"}."Close Display" -> [w446]
    tunnel: w13 -> [w444]
    tunnel: w15 -> [w445]
    tunnel: [w442] -> w7
    shift-right: [w441] -> w5
    shift-left: w14 -> [w443]
    i -> [w448]
    stop <- w449 stop-if-true
    n156 = case shown="\"Close Display\"" w446 {
      tunnel: [w451 w459] -> w442
      tunnel: [w450 w458] -> w441
      tunnel: [w452 _] -> _
      tunnel: w445 -> [w451 w459]
      tunnel: w444 -> [w452 w456]
      tunnel: w443 -> [w450 w458]
      frame "Close Display" {
        n157 = disable-structure shown="RUN_TIME_ENGINE==True" {
          frame condition #0 (active) {
          }
          frame condition #1 {
            n158 = control-ref of="This VI"() -> (w453:refnum<vi>)
            n159 = invoke class="VI" method="FP.Open"(reference=w453, "Activate"=TRUE ("Activate?"), "State"=T10."Hidden") -> ()  [unwired: 2 in, 5 out]
          }
        }
      }
      frame "Clear References" {
        n160 = Unbundle By Name(w458) -> ("Framework Data.Exit Event"=w457:T5)
        n161 = Unregister For Events(event registration refnum=w456) -> ()  [unwired: 1 in, 1 out]
        n162 = Destroy User Event(user event=w457) -> ()  [unwired: 1 in, 1 out]
      }
    }
    n163 = call "Enum Loop Complete.vi"("Current State Enum"=w446, "Itteration"=w448) -> ("Loop Complete?"=w449:bool)  [unwired: 13 out]
    n164 = Increment(x=w446) -> (x+1=w447:enum16{"Close Display", "Clear References"})
  }
  n165 = Unbundle By Name(w5) -> ("Framework Data.Terminate Error"=w3:errorcluster)
  n166 = disable-structure shown="RUN_TIME_ENGINE==True" {
    disable-tunnel: [w460 w461] -> w4
    disable-tunnel: w7 -> [w460 w461]
    frame condition #0 (active) {
    }
    frame condition #1 {
      n167 = Quit LabVIEW() -> ()  [unwired: 1 in]
    }
  }
  n168 = Merge Errors(w3, w4) -> (→"error out":errorcluster)
